vi "Delay over UDP(Rx).vi"() -> ()   [LabVIEW 2014]
panel:
  in  "remote port":u16=54322
  in  "stop":bool
  out "error out":errorcluster
  in  "IP Address":string="192.168.1.101"
  in  "local port":u16=54321
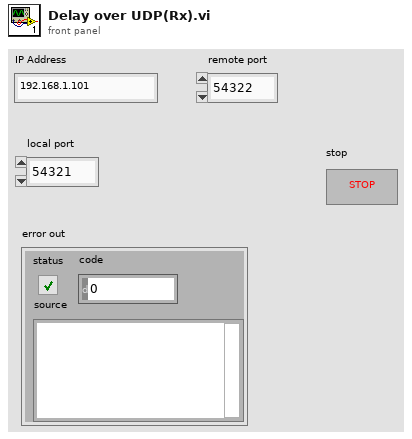
[diagram p1: front panel]
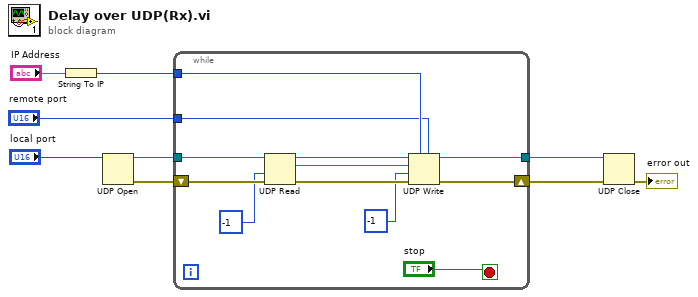
[diagram p0: block diagram]
diagram:
  n1 = String To IP(1:"IP Address") -> (0:w4:u32)
  n2 = UDP Open(11:"local port") -> (port=w8:refnum<k16>, 0:w6:errorcluster)  [unwired: 4 in, 1 out]
  n3 = while {
    tunnel: w4 -> [w14]
    shift-right: [w16] -> w5
    shift-left: w6 -> [w18]
    tunnel: w8 -> [w21]
    tunnel: [w19] -> w7
    tunnel: "remote port" -> [w10]
    stop <- "stop" stop-if-true
    n4 = UDP Read(connection ID=w21, timeout ms (25000)=-1, 8:w18) -> (data out=w13:string, error out=w17:errorcluster, 3:w20:refnum<k16>)  [unwired: 1 in, 2 out]
    n5 = UDP Write(address=w14, port or service name=w10, connection ID=w20, data in=w13, 8:w17, 9:-1 ("timeout ms (25000)")) -> (error out=w16:errorcluster, 3:w19:refnum<k16>)
  }
  n6 = UDP Close(connection ID=w7, 8:w5) -> (error out=→"error out":errorcluster)  [unwired: 1 out]
